vi "Close.vi"(8 "error in (no error)":errorcluster, 11 "VISA Stream in":refnum<class "Serial Stream.lvclass">) -> (0 "error out":errorcluster, 3 "VISA Stream out":refnum<class "Serial Stream.lvclass">)   [LabVIEW 2020, in "Stream-Serial.lvlib" / "Serial Stream.lvclass"]
doc: "Closes the stream after which no more data can be read or written. This will put the connection instance back into an Idle state and it can be opened again when desired."
uses:
  Serial Stream.lvclass
  Client Command.ctl
  Serial Stream.lvclass/Serial Stream.ctl
  Stream-Serial.lvlib
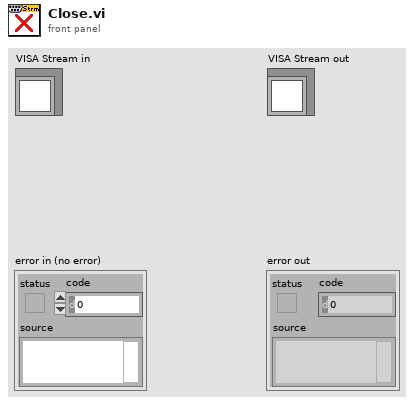
[diagram p1: front panel]
types:
  T1 = typedef "Stream-Serial.lvlib/Client Command.ctl" = enum16{"Connect", "Close", "Shutdown", "Reconnect"}
  T2 = typedef "Stream-Serial.lvlib/Serial Stream.lvclass/Ref Data.ctl" = cluster{"Command Queue":T3}
  T3 = typedef "Stream-Serial.lvlib/Command Queue.ctl" = refnum<queue>
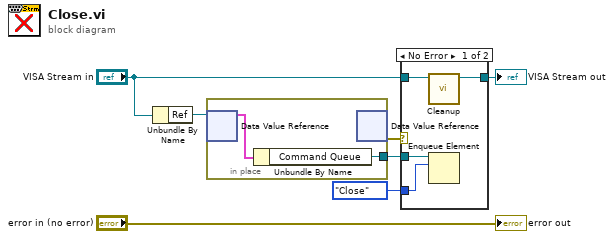
[diagram p0: block diagram]
diagram:
  n1 = Unbundle By Name("VISA Stream in") -> ("Ref"=w6:refnum<data-value>)
  n2 = in-place {
    in-place-border: [w8] -> w5
    n3 = in-place-dvr #1(w6) -> (w9:T2)  [unwired: 1 out]
    n4 = Unbundle By Name(w9) -> ("Command Queue"=w8:T3)
    n5 = in-place-dvr #1() -> (w4:errorcluster)  [unwired: 1 in, 1 out]
  }
  n6 = case shown="No Error" w4 {
    tunnel: w5 -> [w11 _]
    tunnel: "VISA Stream in" -> [w13 w14]
    tunnel: [w12 w14] -> w2
    tunnel: Client_Command."Close" ("Command") -> [w10 _]
    frame No Error {
      n7 = call "Cleanup.vi"("Serial Stream in"=w13) -> ("Serial Stream out"=w12:refnum<class "Serial Stream.lvclass">)  [unwired: 9 in, 1 out]
      n8 = Enqueue Element(queue=w11, element=w10) -> ()  [unwired: 2 in, 3 out]
    }
    frame Error {
    }
  }
  "VISA Stream out" <- w2
  "error out" <- "error in (no error)"
